vi "System Init.vi"(8 "error in (no error)":errorcluster) -> (0 "error out":errorcluster, 3 "qbus out":refnum<class "Qbus.lvclass">)   [LabVIEW 2015, in "Exposure Process.lvlib"]
uses:
  Exposure Process.lvlib
  <vilib>/addons/Qbus/Qbus.lvclass
  FileHandler/FileHandler.lvlib
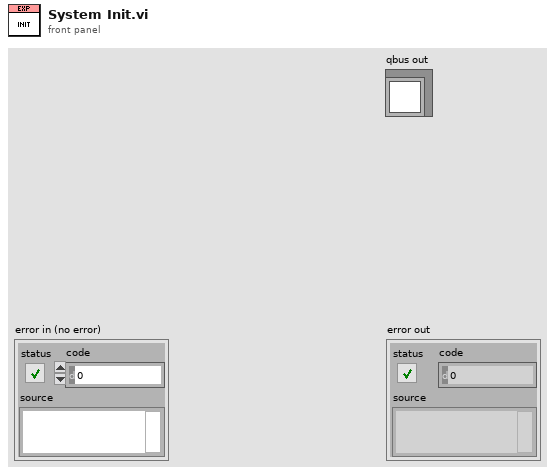
[diagram p1: front panel]
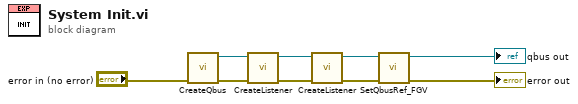
[diagram p0: block diagram]
diagram:
  n1 = call <vilib>:"CreateQbus.vi"("error in (no error)"="error in (no error)") -> ("error out"=w8:errorcluster, "Qbus"=w9:refnum<class "Qbus.lvclass">)  [unwired: 9 in]
  n2 = call "CreateListener.vi"("error in (no error)"=w8, "qbus in"=w9) -> ("error out"=w5:errorcluster, "qbus out"=w6:refnum<class "Qbus.lvclass">)  [unwired: 8 in]
  n3 = call "CreateListener.vi"("error in (no error)"=w5, "qbus in"=w6) -> ("error out"=w4:errorcluster, "qbus out"=w3:refnum<class "Qbus.lvclass">)  [unwired: 8 in]
  n4 = call <vilib>:"SetQbusRef_FGV.vi"("error in (no error)"=w4, "Qbus in"=w3) -> ("error out"=→"error out":errorcluster, "Qbus out"=→"qbus out":refnum<class "Qbus.lvclass">)  [unwired: 8 in]
